vi "_Test - Set Graph Size.vi"() -> ()   [LabVIEW 2024, in "EQMF.lvlib" / "Controls.lvlib"]
uses:
  Controls.lvlib
panel:
  in  "Aspect Ratio":cluster{"W/H":dbl, "Enable":bool}={"W/H"=1.0, "Enable"=FALSE} {"W/H" format="%.2g"}
  in  "Min Size":cluster{"Width":i32, "Height":i32}={"Width"=250, "Height"=200}
  out "error out":errorcluster
  in  "dY":i32
  in  "dX":i32
  in  "Tab Control":enum32{"Page 1", "Page 2"}(tab)
  out "Signal Strength Graph":cluster{"Time":timestamp[], "Link":dbl[]}[](graph) caption="GPS Satellites"
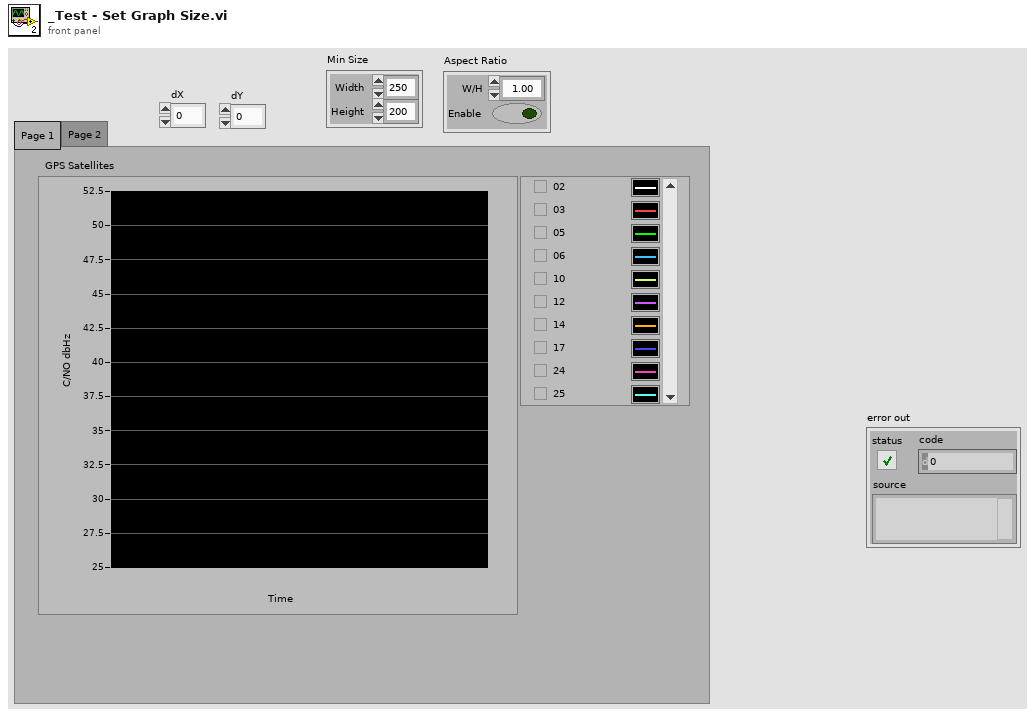
[diagram p1: front panel]
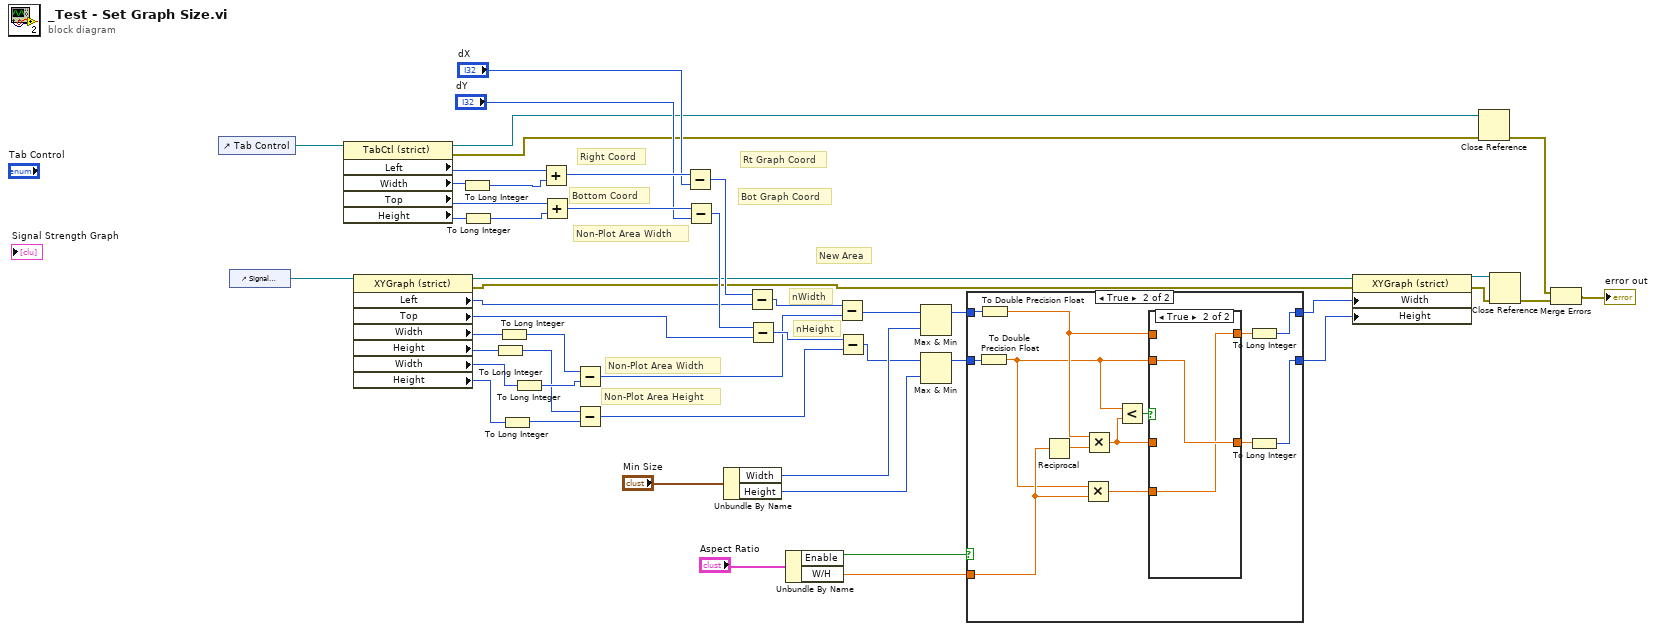
[diagram p0: block diagram]
diagram:
  # "nHeight"
  # "nWidth"
  # "New Area"
  # "Bot Graph Coord"
  # "Rt Graph Coord"
  # "Non-Plot Area Width"
  # "Bottom Coord"
  # "Right Coord"
  # "Non-Plot Area Height"
  # "Non-Plot Area Width"
  n1 = control-ref of="Tab Control"() -> (w41:refnum<vi>)
  n2 = control-ref of="Signal Strength Graph"() -> (w42:refnum<vi>)
  n3 = property on="Property Node" class="TabCtl (strict)"(reference=w41) -> (reference out=w20:refnum<vi>, error out=w19:errorcluster, "Left"=w35:i32, "Width"=w38:u32, "Top"=w36:i32, "Height"=w37:u32)  [unwired: 1 in]
  n4 = property on="Property Node" class="XYGraph (strict)"(reference=w42) -> (reference out=w21:refnum<vi>, error out=w18:errorcluster, "Left"=w27:i32, "Top"=w26:i32, "Width"=w34:u32, "Height"=w49:u32, "Width"=w48:u32, "Height"=w47:u32)  [unwired: 1 in]
  n5 = To Long Integer(number=w38) -> (32bit integer=w39:i32)
  n6 = To Long Integer(number=w37) -> (32bit integer=w40:i32)
  n7 = To Long Integer(number=w49) -> (32bit integer=w44:i32)
  n8 = To Long Integer(number=w34) -> (32bit integer=w45:i32)
  n9 = To Long Integer(number=w47) -> (32bit integer=w43:i32)
  n10 = To Long Integer(number=w48) -> (32bit integer=w46:i32)
  n11 = Add(x=w35, y=w39) -> (x+y=w32:i32)
  n12 = Add(x=w36, y=w40) -> (x+y=w33:i32)
  n13 = Subtract(x=w45, y=w46) -> (x-y=w23:i32)
  n14 = Subtract(x=w44, y=w43) -> (x-y=w22:i32)
  n15 = Subtract(x=w32, y="dX") -> (x-y=w29:i32)
  n16 = Subtract(x=w33, y="dY") -> (x-y=w28:i32)
  n17 = Unbundle By Name("Min Size") -> ("Width"=w11:i32, "Height"=w10:i32)
  n18 = Subtract(x=w29, y=w27) -> (x-y=w25:i32)
  n19 = Subtract(x=w28, y=w26) -> (x-y=w24:i32)
  n20 = Unbundle By Name("Aspect Ratio") -> ("Enable"=w2:bool, "W/H"=w1:dbl)
  n21 = Subtract(x=w25, y=w23) -> (x-y=w8:i32)
  n22 = Subtract(x=w24, y=w22) -> (x-y=w9:i32)
  n23 = Max & Min(x=w8, y=w11) -> (max(x,y)=w7:i32)  [unwired: 1 out]
  n24 = Max & Min(x=w9, y=w10) -> (max(x,y)=w6:i32)  [unwired: 1 out]
  n25 = case shown="True" w2 {
    tunnel: w7 -> [w51 w64]
    tunnel: w6 -> [w50 w63]
    tunnel: [w51 w55] -> w5
    tunnel: [w50 w56] -> w4
    tunnel: w1 -> [_ w61]
    frame False {
    }
    frame True {
      n26 = To Double Precision Float(number=w63) -> (double precision float=w53:dbl)
      n27 = To Double Precision Float(number=w64) -> (double precision float=w60:dbl)
      n28 = Reciprocal(x=w61) -> (1/x=w62:dbl)
      n29 = Multiply(x=w53, y=w61) -> (x*y=w52:dbl)
      n30 = Multiply(x=w60, y=w62) -> (x*y=w59:dbl)
      n31 = Less?(x=w53, y=w59) -> (x < y?=w58:bool)
      n32 = case shown="True" w58 {
        tunnel: w60 -> [w66 _]
        tunnel: w59 -> [w65 _]
        tunnel: [w66 w67] -> w54
        tunnel: [w65 w68] -> w57
        tunnel: w53 -> [_ w68]
        tunnel: w52 -> [_ w67]
        frame False {
        }
        frame True {
        }
      }
      n33 = To Long Integer(number=w54) -> (32bit integer=w55:i32)
      n34 = To Long Integer(number=w57) -> (32bit integer=w56:i32)
    }
  }
  n35 = property on="Property Node" class="XYGraph (strict)"(reference=w21, error in=w18, "Width"=w5, "Height"=w4) -> (reference out=w17:refnum<vi>, error out=w16:errorcluster)
  n36 = Close Reference(reference=w20, error in (no error)=w19) -> (error out=w14:errorcluster)
  n37 = Close Reference(reference=w17, error in (no error)=w16) -> (error out=w15:errorcluster)
  n38 = Merge Errors(w14, w15) -> (→"error out":errorcluster)
